vi "Appply Application Style.vi"(8 "error in (no error)":errorcluster, 10 "VI Refnum":refnum<vi>, 11 "IApplicationStyle in":refnum<class "IApplicationStyle.lvclass">) -> (0 "error out":errorcluster)   [LabVIEW 2015, in "IViewable.lvlib" / "IApplicationStyle.lvclass"]
uses:
  IApplicationStyle.lvclass
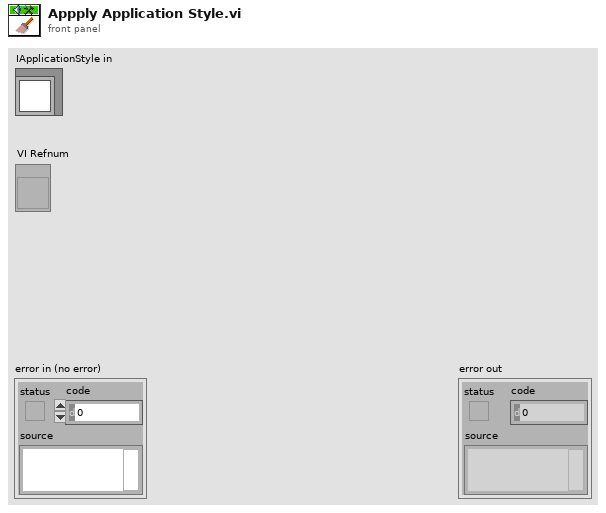
[diagram p1: front panel]
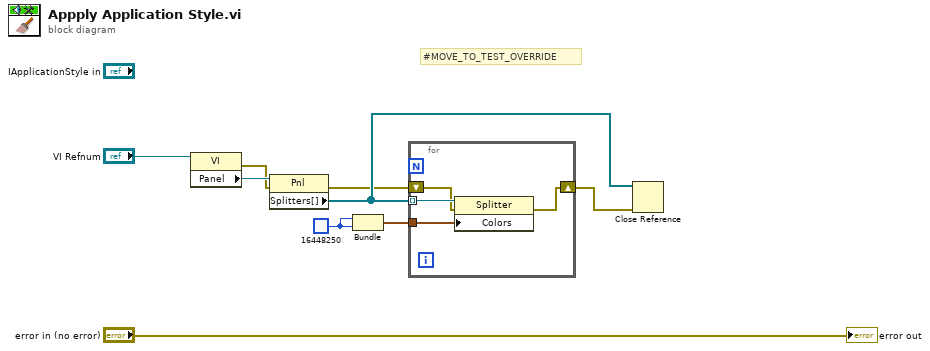
[diagram p0: block diagram]
diagram:
  w6 = u32 16448250
  # "#MOVE_TO_TEST_OVERRIDE"
  n1 = property class="VI"(reference="VI Refnum") -> (error out=w3:errorcluster, "Panel"=w7:refnum<vi>)  [unwired: 1 in, 1 out]
  n2 = property class="Pnl"(reference=w7, error in=w3) -> (error out=w2:errorcluster, "Splitters[]"=w4:refnum<vi>[])  [unwired: 1 out]
  n3 = Bundle(w6, w6) -> (w5:cluster{u32, u32})  [unwired: 1 in]
  n4 = for {
    tunnel: w4 -> [w13] mode=indexing
    tunnel: w5 -> [w12]
    shift-right: [w10] -> w1
    shift-left: w2 -> [w11]
    n5 = property class="Splitter"(reference=w13, error in=w11, "Colors"=w12) -> (error out=w10:errorcluster)  [unwired: 1 out]
  }
  n6 = Close Reference(reference=w4, error in (no error)=w1) -> ()  [unwired: 1 out]
  "error out" <- "error in (no error)"
